vi "Launch Threads.vi"(7 "options":T1, 8 "error in (no error)":errorcluster, 10 "Threads":refnum<class "Thread.lvclass">[](array[class]), 11 "Framework in":refnum<class "Framework.lvclass">) -> (0 "error out":errorcluster, 3 "Framework out":refnum<class "Framework.lvclass">)   [LabVIEW 2017, in "DSF Core.lvlib" / "Framework.lvclass"]
uses:
  Framework.lvclass
  Thread/Thread.lvclass
  Thread/Thread Options.ctl
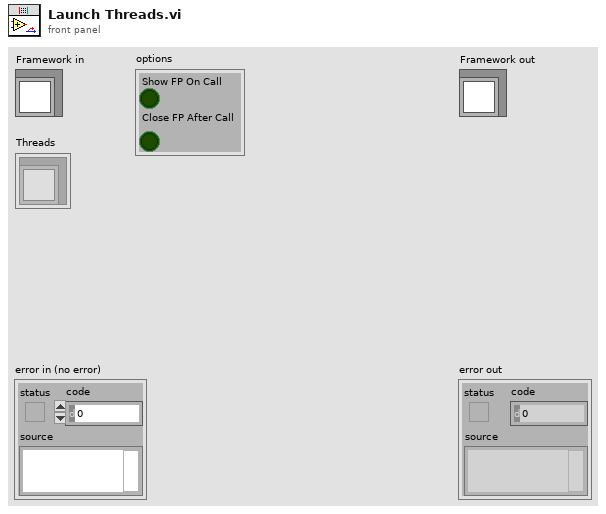
[diagram p1: front panel]
types:
  T1 = typedef "DSF Core.lvlib/Thread.lvclass/Thread Options.ctl" = cluster{"Show FP On Call":bool, "Close FP After Call":bool}
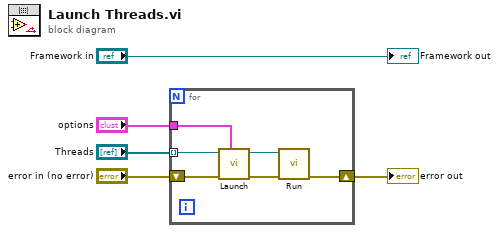
[diagram p0: block diagram]
diagram:
  n1 = for {
    shift-right: [w6] -> w1
    shift-left: "error in (no error)" -> [w11]
    tunnel: "Threads" -> [w10] mode=indexing
    tunnel: "options" -> [w9]
    n2 = call "Launch.vi"("options"=w9, "error in (no error)"=w11, "Thread in"=w10) -> ("error out"=w7:errorcluster, "Thread out"=w8:refnum<class "Thread.lvclass">)  [unwired: 7 in]
    n3 = call "Run.vi"("error in (no error)"=w7, "Thread in"=w8) -> ("error out"=w6:errorcluster)  [unwired: 8 in, 1 out]
  }
  "error out" <- w1
  "Framework out" <- "Framework in"
